vi "Get Target Time Elapsed Event.vi"(8 "error in (no error)":errorcluster, 11 "Timer in":refnum<class "Timer.lvclass">) -> (0 "error out":errorcluster, 2 "Target Time Elapsed Event":refnum<user-event>, 3 "Timer out":refnum<class "Timer.lvclass">)   [LabVIEW 2018, in "Timer.lvclass"]
uses:
  Timer.lvclass
  Timer.lvclass/Timer.ctl
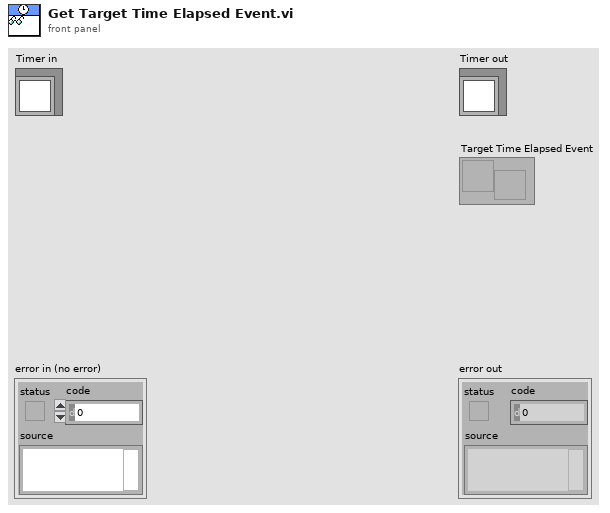
[diagram p1: front panel]
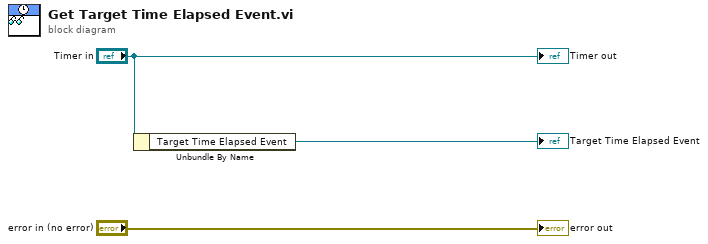
[diagram p0: block diagram]
diagram:
  n1 = Unbundle By Name("Timer in") -> ("Target Time Elapsed Event"=→"Target Time Elapsed Event":refnum<user-event>)
  "error out" <- "error in (no error)"
  "Timer out" <- "Timer in"
